vi "MAIN - Create New REx_CMD.vi"() -> ()   [LabVIEW 2012, in "REx_Springboard.lvlib"]
uses:
  _CMD_Springboard/REx_Springboard.lvlib
  _CMD_Springboard/Dependencies.llb/Exit Req Event Registration Ref.ctl
  <vilib>/LabVIEW Icon API/API_Text.ctl
  <vilib>/LabVIEW Icon API/API_User Layer Data.ctl
  <vilib>/Utility/miscctls.llb/LVPoint32TypeDef.ctl
  <vilib>/picture/picture.llb/imagedata.ctl
  <vilib>/LabVIEW Icon API/API_Test Settings.ctl
  <vilib>/LabVIEW Icon API/lv_icon/Controls/Alignment.ctl
  <vilib>/LabVIEW Icon API/API_Text Colors.ctl
  <vilib>/Utility/error.llb/DialogTypeEnum.ctl
  _CMD_Springboard/TypeDef - SHIFTER - GUI Template.ctl
  _CMD_Springboard/Dependencies.llb/TLB_Dependencies.lvlib
  <vilib>/LabVIEW Icon API/LabVIEW Icon API.lvlib
panel:
  out "Icon Preview":picture
  in  "Wait For Response?":bool=TRUE
  in  "Timeout, ms":i32=-1
  in  "Line 2 text":string
  in  "Line 1 text":string
  in  "Add to Project":u16(ring) items=["REx.lvproj", "Untitled Project 1", "< Create In New Project... >"]
  in  "Cancel":bool
  in  "Build":bool
  in  "New Command Name":string
  in  "Destination Folder":path
  out "error out":errorcluster
  # "New REx CMD"
  # "Description"
  # "Configuration"
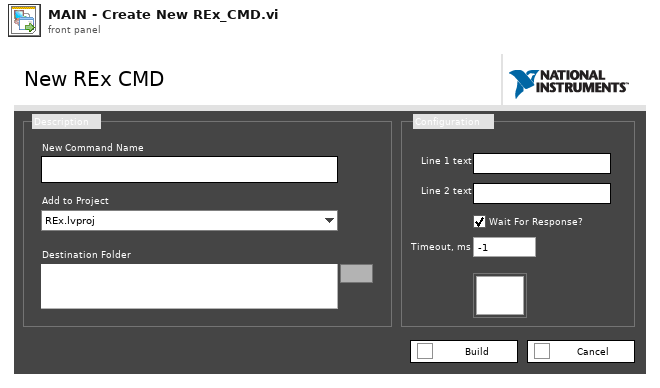
[diagram p1: front panel]
types:
  T1 = enum16{"Clear SR", "Set Display", "Set Shifter", "Initialize Events", "Init Q"}
  T2 = typedef "REx_Springboard.lvlib/TypeDef - SHIFTER - GUI Template.ctl" = cluster{"Exit Event":T3, "Terminate Error":errorcluster, "User Parameter Controls":refnum<vi>[], "User Parameters":cluster{"New REx Name":string, "Destination Folder":path, "Project Selection":u16, "Line 1 text":string, "Line 2 text":string, "Timeout":i32, "Wait For Response?":bool}, "Display Data":cluster{"Copy Successful?":bool}, "Projects In Memory":refnum<vi>[], "New Library Path":path, "Template Library Path":path, "Template Class Reference":refnum<vi>, "Selected Project":refnum<vi>}
  T3 = typedef "REx_Springboard.lvlib/TLB_Dependencies.lvlib/Exit Event Ref.ctl" = refnum<user-event>
  T4 = typedef "REx_Springboard.lvlib/TLB_Dependencies.lvlib/Exit Req Event Registration Ref.ctl" = refnum<event-registration>
  T5 = cluster{"Event Registration Refnum":refnum<event-registration>, "Exit Req Event Registration Ref":T4}
  T6 = typedef "REx_Springboard.lvlib/TLB_Dependencies.lvlib/amc_Message Queue.ctl" = refnum<queue>
  T7 = typedef "LabVIEW Icon API.lvlib/API_User Layer Data.ctl" = cluster{"Layer name":string, "Origin":T8, "Icon image data":T9}
  T8 = typedef "LVPoint32TypeDef.ctl" = cluster{"Horizontal":i32, "Vertical":i32}
  T9 = typedef "imagedata.ctl" = cluster{"image type":i32, "image depth":i32, "image":u8[], "mask":u8[], "colors":u32[], "Rectangle":cluster{"left":i16, "top":i16, "right":i16, "bottom":i16}}
  T10 = typedef "LabVIEW Icon API.lvlib/API_Text.ctl" = cluster{"Line 1 text":string, "Line 2 text":string, "Line 3 text":string, "Line 4 text":string}
  T11 = typedef "DialogTypeEnum.ctl" = enum16{"no dialog", "OK message", "continue or stop message", "auto error handling dialog", "OK message + warnings", "continue/stop + warnings"}
  T12 = typedef "LabVIEW Icon API.lvlib/API_Test Settings.ctl" = cluster{"Font":string, "Alignment":T13, "Size":u8, "Center text":bool, "Capitalize text":bool, "Text color":T14}
  T13 = typedef "Alignment.ctl" = u16
  T14 = typedef "LabVIEW Icon API.lvlib/API_Text Colors.ctl" = cluster{"Line 1 color":u32, "Line 2 color":u32, "Line 3 color":u32, "Line 4 color":u32}
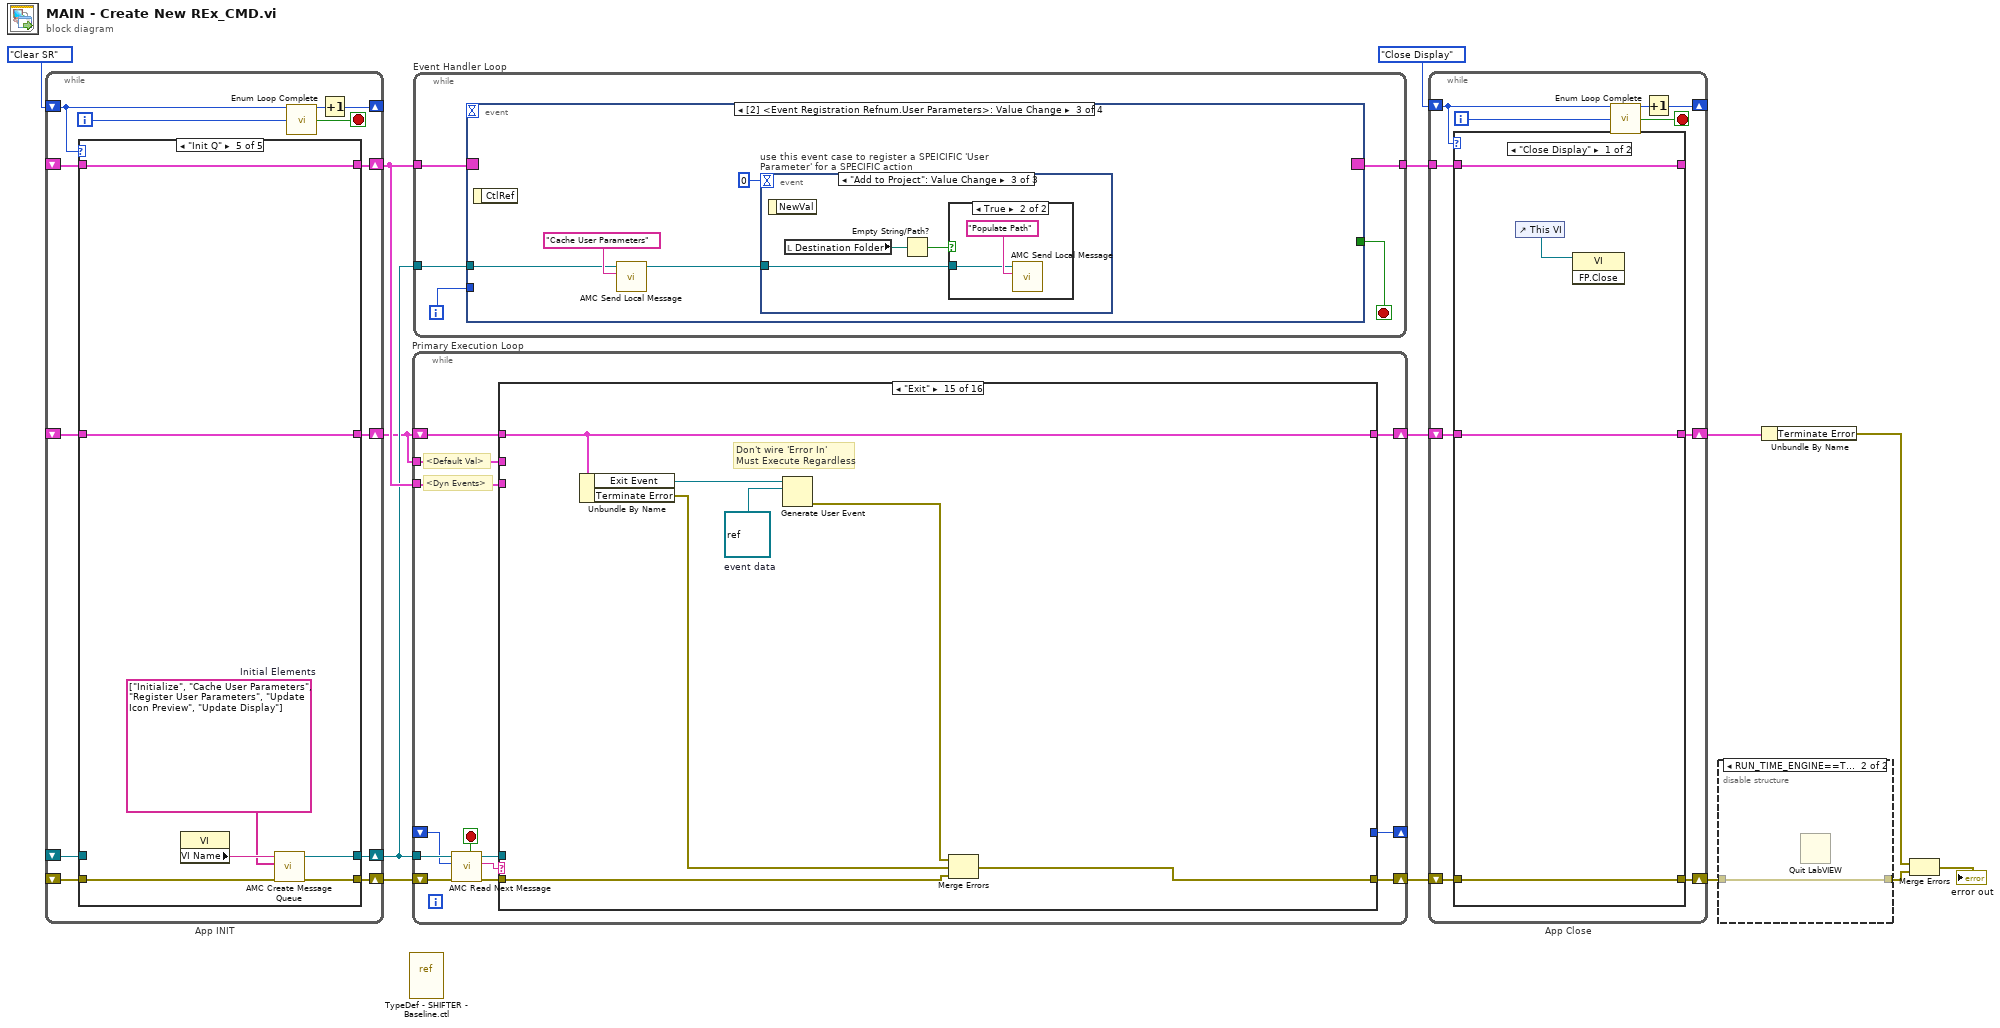
[diagram p0: block diagram]
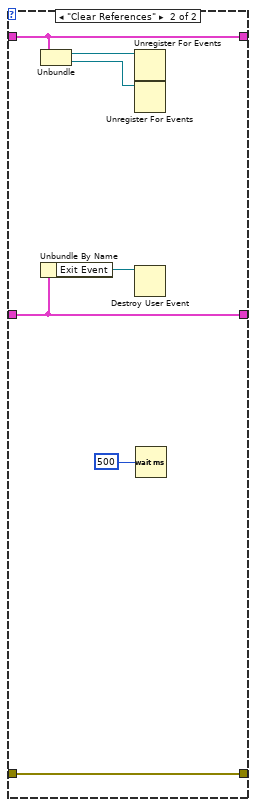
[diagram p3: hidden frame]
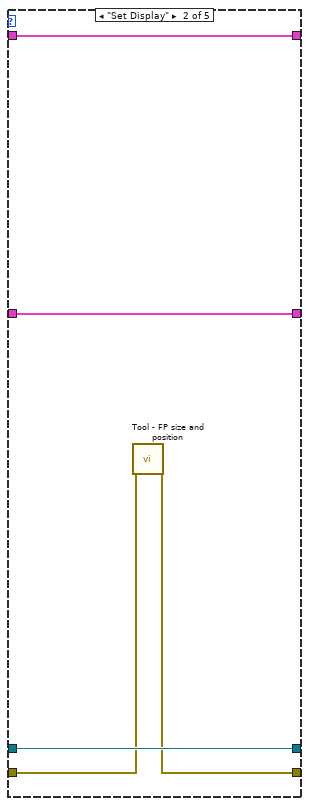
[diagram p5: hidden frame]
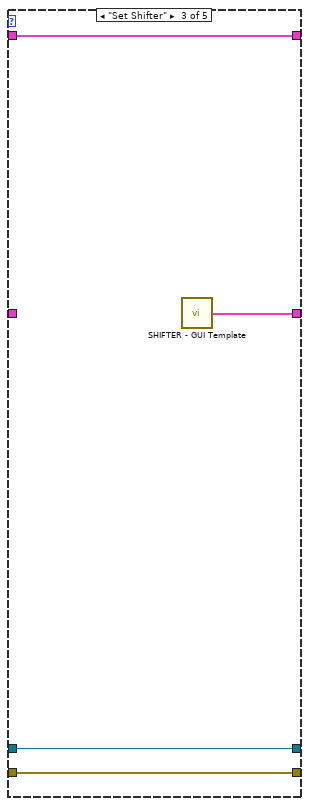
[diagram p6: hidden frame]
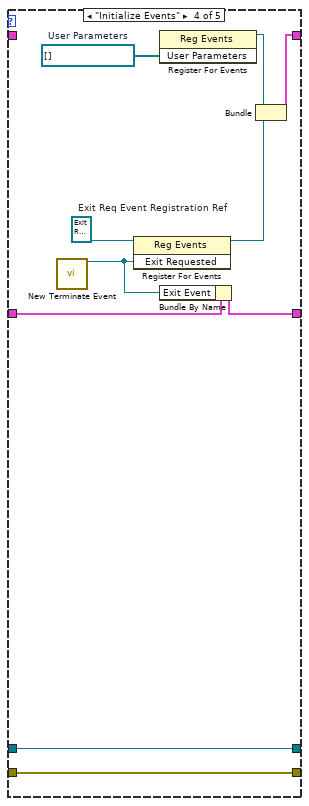
[diagram p7: hidden frame]
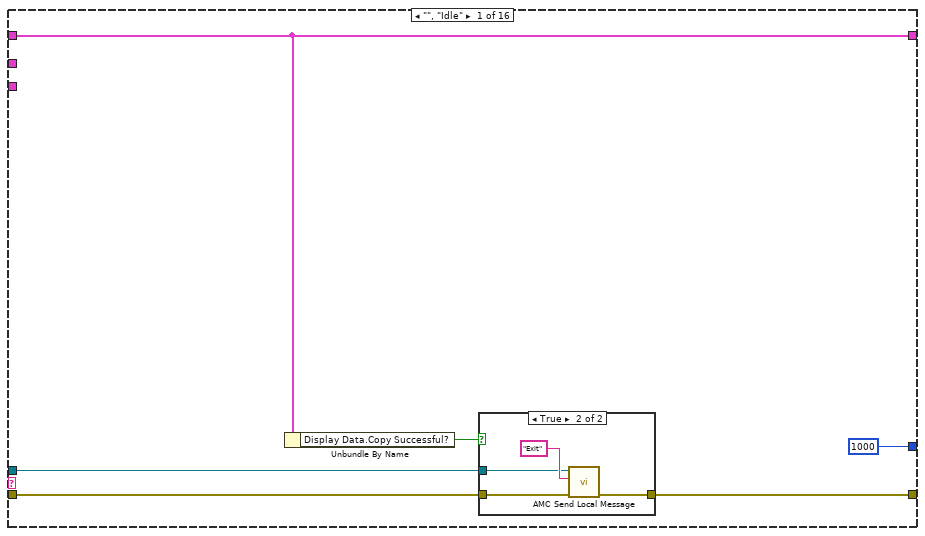
[diagram p8: hidden frame]
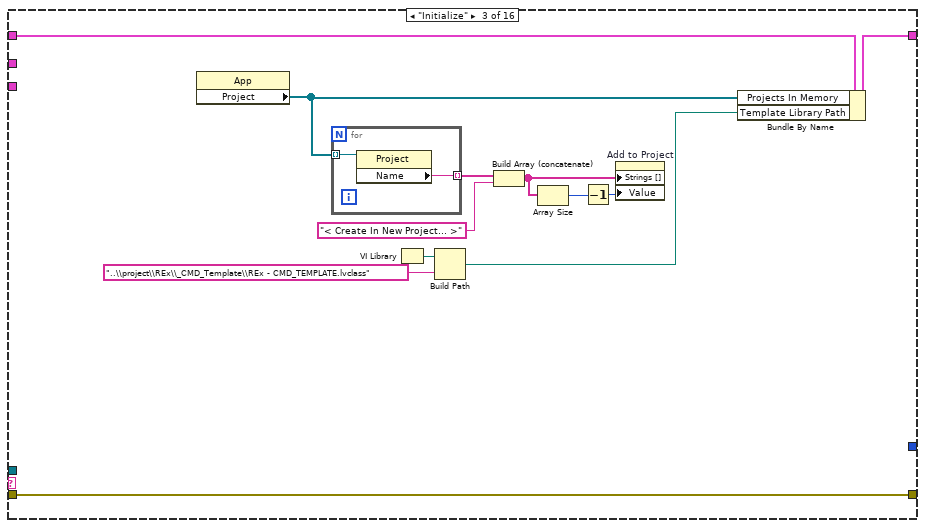
[diagram p11: hidden frame]
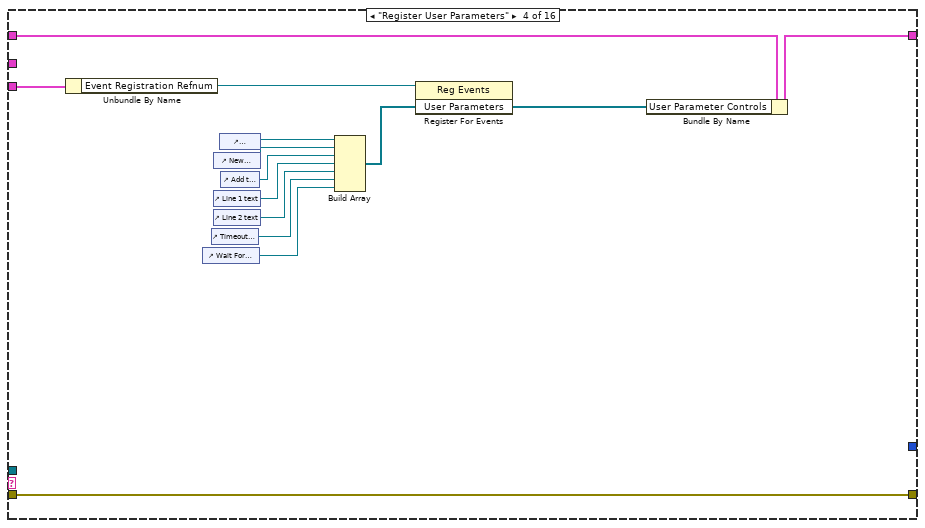
[diagram p12: hidden frame]
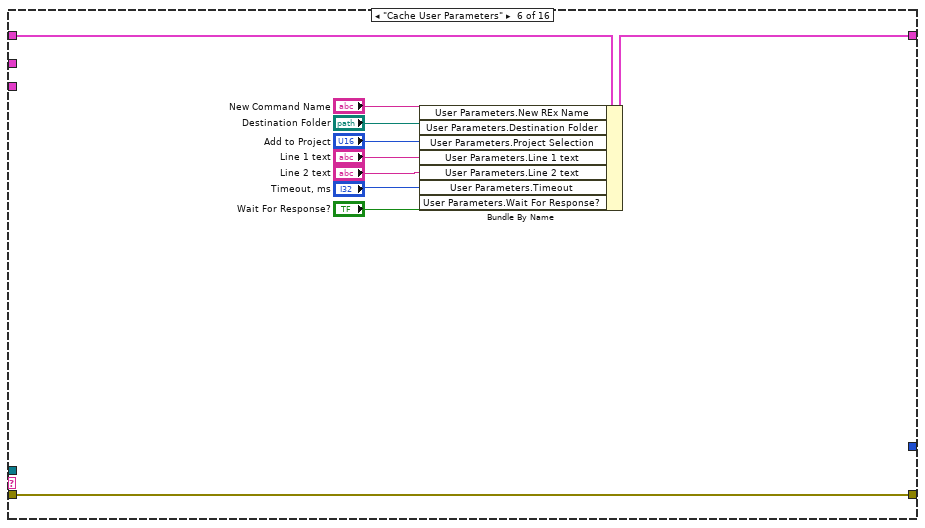
[diagram p14: hidden frame]
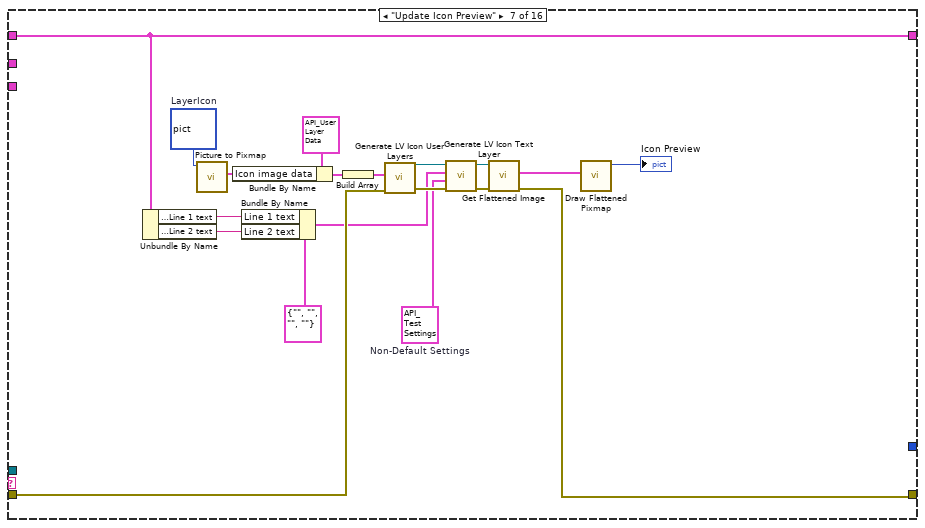
[diagram p15: hidden frame]
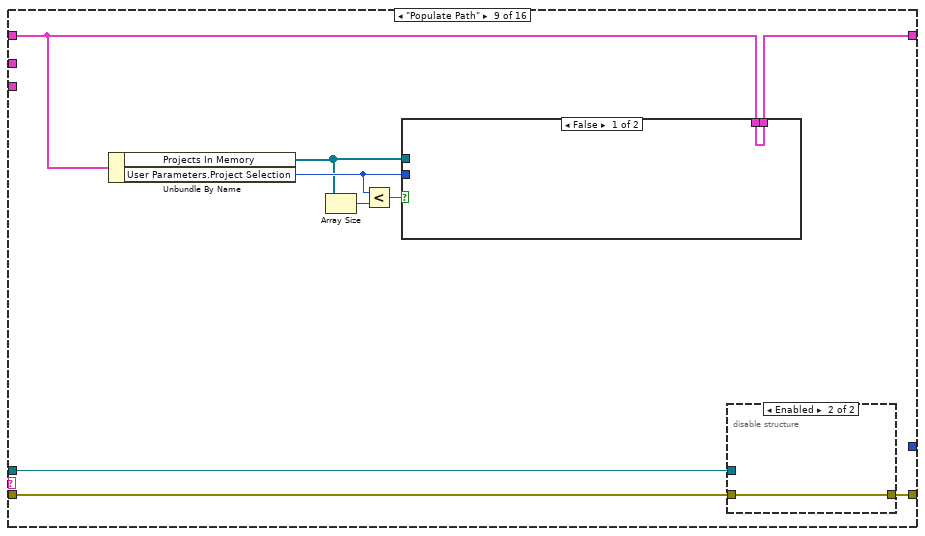
[diagram p17: hidden frame]
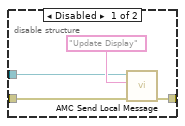
[diagram p18: hidden frame]
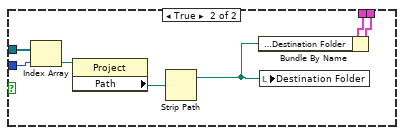
[diagram p19: hidden frame]
diagram:
  n1 = while "App INIT" {
    shift-right: [w20] -> _
    shift-left: T1."Clear SR" -> [w15]
    shift-right: [w26] -> w8
    shift-left: _ -> [w19]
    shift-right: [w23] -> w7
    shift-left: _ -> [w18]
    shift-right: [w25] -> w10
    shift-left: _ -> [w17]
    shift-right: [w24] -> w6
    shift-left: _ -> [w16]
    i -> [w21]
    stop <- w22 stop-if-true
    n2 = case shown="\"Init Q\"" w15 {
      tunnel: [w28 w31 w36 w47 w51] -> w26
      tunnel: [w27 w29 w35 w46 w49] -> w23
      tunnel: [_ w33 w37 w39 w53] -> w24
      tunnel: [_ w32 w34 w44 w54] -> w25
      tunnel: w19 -> [w28 w31 w36 w47 _]
      tunnel: w18 -> [w27 w30 w35 w46 w50]
      tunnel: w17 -> [_ w32 w34 _ w54]
      tunnel: w16 -> [_ w33 _ w40 w53]
      frame "Clear SR" {
      }
      frame "Set Display" {
        n3 = call "Tool - FP size and position.vi"("error in (no error)"=w30) -> ("error out"=w29:errorcluster)  [unwired: 7 in, 11 out]
      }
      frame "Set Shifter" {
        n4 = call "SHIFTER - GUI Template.vi"() -> ("SHIFTER DATA"=w37:T2)  [unwired: 15 out]
      }
      frame "Initialize Events" {
        w41 = T4 refnum  # Exit Req Event Registration Ref
        w45 = refnum<vi>[] []  # User Parameters
        n5 = call "New Terminate Event.vi"() -> ("Exit Event Ref"=w38:T3)  [unwired: 13 in, 2 out]
        n6 = register-events(reference=w41, w38) -> (reference out=w42:T4)  [unwired: 1 in, 1 out]
        n7 = register-events(w45) -> (reference out=w43:refnum<event-registration>)  [unwired: 2 in, 1 out]
        n8 = Bundle By Name(cluster=w40, "Exit Event"=w38) -> (w39:T2)
        n9 = Bundle("Event Registration Refnum"=w43, "Exit Req Event Registration Ref"=w42) -> (w44:T5)  [unwired: 1 in]
      }
      frame "Init Q" {
        w48 = string[] ["Initialize", "Cache User Parameters", "Register User Parameters", "Update Icon Preview", "Update Display"]  # Initial Elements
        n10 = property class="VI"() -> ("VI Name"=w52:string)  [unwired: 2 in, 2 out]
        n11 = call "AMC Create Message Queue.vi"("error in (no error)"=w50, "Initial Message Names"=w48, "Message Queue Name"=w52) -> ("error out"=w49:errorcluster, "Message Queue out"=w51:T6)  [unwired: 7 in]
      }
    }
    n12 = call "Enum Loop Complete.vi"("Current State Enum"=w15, "Itteration"=w21) -> ("Loop Complete?"=w22:bool)  [unwired: 13 out]
    n13 = Increment(x=w15) -> (x+1=w20:T1)
  }
  n14 = vi-ref "TypeDef - SHIFTER - Baseline.ctl"() -> ()  [unwired: 1 out]
  n15 = while "Primary Execution Loop" {
    shift-right: [w67] -> w14
    shift-left: w7 -> [w59]
    shift-right: [w64] -> _
    shift-left: _ -> [w56]
    shift-right: [w63] -> w13
    shift-left: w6 -> [w66]
    tunnel: w6 -> [w65]
    tunnel: w8 -> [w61]
    tunnel: w10 -> [w62]
    stop <- w57 stop-if-true
    # "<Dyn Events>"
    # "<Default Val>"
    n16 = call "AMC Read Next Message.vi"("error in (no error)"=w59, "timeout (1ms)"=w56, "Message Queue in"=w61) -> ("error out"=w58:errorcluster, "Message Name"=w55:string, "Message Queue out"=w60:T6, "Exit Process"=w57:bool)  [unwired: 2 in, 3 out]
    n17 = case shown="\"Exit\"" w55 {
      selector: w55 -> [_ _ _ _ _ _ _ _ _ _ _ _ _ _ _ w237]
      tunnel: [w70 w80 w84 w107 w109 w117 w132 w140 w147 w164 w168 w204 w207 w214 w232 w241] -> w67
      tunnel: w58 -> [w71 w80 w84 w107 w109 w117 w138 w140 w148 w164 w172 w188 w207 w216 w230 w242]
      tunnel: w60 -> [w68 _ _ _ _ _ _ _ w149 _ _ _ _ w212 _ _]
      tunnel: w66 -> [w72 w79 w92 w106 w108 w119 w135 w139 w142 w163 w176 w196 w206 w209 w235 w243]
      tunnel: w65 -> [_ _ _ _ _ _ _ _ _ _ _ _ _ _ _ _]
      tunnel: [w72 w79 w91 w105 w108 w118 w135 w139 w141 w163 w175 w196 w206 w208 w235 w243] -> w63
      tunnel: [1000 _ _ _ _ _ _ _ _ _ _ _ _ _ _ _] -> w64
      tunnel: w62 -> [_ _ _ w104 _ _ _ _ _ _ _ _ _ _ _ _]
      frame "", "Idle" {
        n18 = Unbundle By Name(w72) -> ("Display Data.Copy Successful?"=w69:bool)
        n19 = case shown="True" w69 {
          tunnel: w71 -> [w74 w77]
          tunnel: [w74 w76] -> w70
          tunnel: w68 -> [_ w75]
          frame False {
          }
          frame True {
            n20 = call "AMC Send Local Message.vi"("error in (no error)"=w77, "Message Name"="Exit" ("event"), "Message Queue in"=w75) -> ("error out"=w76:errorcluster)  [unwired: 7 in, 1 out]
          }
        }
      }
      frame "/*********Initialize********/" {
      }
      frame "Initialize" {
        n21 = property class="App"() -> ("Project"=w90:refnum<vi>[])  [unwired: 2 in, 2 out]
        n22 = for {
          tunnel: w90 -> [w94] mode=indexing
          tunnel: [w93] -> w89 mode=indexing
          n23 = property class="Project"(reference=w94) -> ("Name"=w93:string)  [unwired: 1 in, 2 out]
        }
        n24 = VI Library() -> (path=w87:path)
        n25 = Build Path(base path=w87, name or relative path="..\\project\\REx\\_CMD_Template\\REx - CMD_TEMPLATE.lvclass") -> (appended path=w85:path)
        n26 = Build Array (concatenate)(w89, "< Create In New Project... >") -> (w83:string[])
        n27 = Array Size(array=w83) -> (size(s)=w82:i32)
        n28 = Decrement(x=w82) -> (x-1=w81:i32)
        n29 = property on="Add to Project" class="Ring (strict)"("Strings []"=w83, "Value"=w81) -> ()  [unwired: 2 in, 2 out]
        n30 = Bundle By Name(cluster=w92, "Projects In Memory"=w90, "Template Library Path"=w85) -> (w91:T2)
      }
      frame "Register User Parameters" {
        n31 = Unbundle By Name(w104) -> ("Event Registration Refnum"=w103:refnum<event-registration>)
        n32 = control-ref of="Wait For Response?"() -> (w95:refnum<vi>)
        n33 = control-ref of="Timeout, ms"() -> (w96:refnum<vi>)
        n34 = control-ref of="New Command Name"() -> (w99:refnum<vi>)
        n35 = control-ref of="Line 1 text"() -> (w98:refnum<vi>)
        n36 = control-ref of="Line 2 text"() -> (w97:refnum<vi>)
        n37 = control-ref of="Destination Folder"() -> (w102:refnum<vi>)
        n38 = control-ref of="Add to Project"() -> (w100:refnum<vi>)
        n39 = Build Array(w102, w99, w100, w98, w97, w96, w95) -> (w101:refnum<vi>[])
        n40 = register-events(reference=w103, w101) -> ()  [unwired: 1 in, 2 out]
        n41 = Bundle By Name(cluster=w106, "User Parameter Controls"=w101) -> (w105:T2)
      }
      frame "/*********Display Updates********/" {
      }
      frame "Cache User Parameters" {
        n42 = Bundle By Name(cluster=w119, "User Parameters.New REx Name"="New Command Name", "User Parameters.Destination Folder"="Destination Folder", "User Parameters.Project Selection"="Add to Project", "User Parameters.Line 1 text"="Line 1 text", "User Parameters.Line 2 text"="Line 2 text", "User Parameters.Timeout"="Timeout, ms", "User Parameters.Wait For Response?"="Wait For Response?") -> (w118:T2)
      }
      frame "Update Icon Preview" {
        w120 = T12 {"Font"="Small Fonts", "Alignment"=1, "Size"=8, "Center text"=FALSE, "Capitalize text"=TRUE, "Text color"={"Line 1 color"=0, "Line 2 color"=0, "Line 3 color"=0, "Line 4 color"=0}}  # Non-Default Settings
        w127 = picture bytes[3230]  # LayerIcon
        n43 = Unbundle By Name(w135) -> ("User Parameters.Line 1 text"=w137:string, "User Parameters.Line 2 text"=w136:string)
        n44 = call <vilib>:"Picture to Pixmap.vi"("picture"=w127) -> ("image data"=w126:T9)  [unwired: 9 in, 1 out]
        n45 = Bundle By Name(cluster=T7 {"Layer name"="", "Origin"={"Horizontal"=0, "Vertical"=0}, "Icon image data"={"image type"=0, "image depth"=0, "image"=[], "mask"=[], "colors"=[], "Rectangle"={"left"=0, "top"=0, "right"=0, "bottom"=0}}} ("User layer"), "Icon image data"=w126) -> (w125:T7)
        n46 = Bundle By Name(cluster=T10 {"Line 1 text"="", "Line 2 text"="", "Line 3 text"="", "Line 4 text"=""} ("Text"), "Line 1 text"=w137, "Line 2 text"=w136) -> (w121:T10)
        n47 = Build Array(w125) -> (w124:T7[])
        n48 = call <vilib>:"Generate LV Icon User Layers.vi"("error in (no error)"=w138, "User layers"=w124) -> ("error out"=w129:errorcluster, "Icon out"=w123:refnum<class "Icon.lvclass">)  [unwired: 8 in]
        n49 = call <vilib>:"Generate LV Icon Text Layer.vi"("error in (no error)"=w129, "Text settings"=w120, "Text"=w121, "Icon in"=w123) -> ("error out"=w131:errorcluster, "Icon out"=w122:refnum<class "Icon.lvclass">)  [unwired: 6 in]
        n50 = call <vilib>:"Get Flattened Image.vi"("error in (no error)"=w131, "lv_icon.lvlib:Icon.lvclass in"=w122) -> ("error out"=w132:errorcluster, "Color Image"=w134:T9)  [unwired: 6 in, 2 out]
        n51 = call <vilib>:"Draw Flattened Pixmap.vi"("image data"=w134) -> ("new picture"=→"Icon Preview":picture)  [unwired: 8 in]
      }
      frame "Update Display" {
      }
      frame "Populate Path" {
        n52 = Unbundle By Name(w142) -> ("Projects In Memory"=w144:refnum<vi>[], "User Parameters.Project Selection"=w146:u16)
        n53 = Array Size(array=w144) -> (size(s)=w145:i32)
        n54 = Less?(x=w146, y=w145) -> (x < y?=w143:bool)
        n55 = case shown="False" w143 {
          tunnel: w146 -> [_ w162]
          tunnel: w144 -> [_ w161]
          tunnel: w142 -> [w155 w159]
          tunnel: [w155 w158] -> w141
          frame False {
          }
          frame True {
            n56 = Index Array(array=w161, index=w162) -> (element=w160:refnum<vi>)
            n57 = property class="Project"(reference=w160) -> ("Path"=w157:path)  [unwired: 1 in, 2 out]
            n58 = Strip Path(path=w157) -> (stripped path=w156:path)  [unwired: 1 out]
            n59 = Bundle By Name(cluster=w159, "User Parameters.Destination Folder"=w156) -> (w158:T2)
            n60 = local write "Destination Folder"(w156) -> ()
          }
        }
        n61 = disable-structure shown="Enabled" {
          disable-tunnel: w149 -> [w152 _]
          disable-tunnel: w148 -> [w151 w154]
          disable-tunnel: [w150 w154] -> w147
          frame Disabled {
            n62 = call "AMC Send Local Message.vi"("error in (no error)"=w151, "Message Name"="Update Display" ("event"), "Message Queue in"=w152) -> ("error out"=w150:errorcluster)  [unwired: 7 in, 1 out]
          }
          frame Enabled {
          }
        }
      }
      frame "/*********Primary Execution********/" {
      }
      frame "Build New CMD" {
        n63 = Unbundle By Name(w176) -> ("Projects In Memory"=w178:refnum<vi>[], "User Parameters.Project Selection"=w180:u16)
        n64 = Unbundle By Name(w176) -> ("Template Library Path"=w166:path, "User Parameters.Destination Folder"=w171:path, "User Parameters.New REx Name"=w170:string)
        n65 = call <vilib>:"Set Busy.vi"("error in (no error)"=w172) -> ("error out"=w169:errorcluster)  [unwired: 9 in, 1 out]
        n66 = Array Size(array=w178) -> (size(s)=w179:i32)
        n67 = Less?(x=w180, y=w179) -> (x < y?=w177:bool)
        n68 = case shown="True" w177 {
          tunnel: w180 -> [_ w185]
          tunnel: w178 -> [_ w184]
          tunnel: [w181 w183] -> w165
          frame False {
            n69 = invoke class="App" method="Project.New"() -> ("Project:New"=w182:refnum<vi>)  [unwired: 3 in, 2 out]
            n70 = invoke class="Project" method="Open Window"(reference=w182) -> (reference out=w181:refnum<vi>)  [unwired: 2 in, 2 out]
          }
          frame True {
            n71 = Index Array(array=w184, index=w185) -> (element=w183:refnum<vi>)
          }
        }
        n72 = call "Copy Library into Project.vi"("Project"=w165, "Library Path"=w166, "Destination Folder"=w171, "New TLB Name"=w170, "error in"=w169) -> ("New Library Path"=w167:path, "error out"=w168:errorcluster)  [unwired: 9 in]
        n73 = Unbundle By Name(w168) -> ("status"=w174:bool)
        n74 = Not(x=w174) -> (.not. x?=w173:bool)
        n75 = Bundle By Name(cluster=w176, "Display Data.Copy Successful?"=w173, "New Library Path"=w167, "Selected Project"=w165) -> (w175:T2)
      }
      frame "Customize CMD" {
        w201 = refnum<vi> refnum  # LVClassLibrary
        # "*Change Event Terminal Names\n*Change Icon\n*Change Short Name\n*Modify Send Command (Wait / Timeout / Direction of Data"
        n76 = Unbundle By Name(w196) -> ("User Parameters.Line 1 text"=w198:string, "User Parameters.Line 2 text"=w197:string, "User Parameters.New REx Name"=w193:string, "Selected Project"=w186:refnum<vi>)
        n77 = Unbundle By Name(w196) -> ("New Library Path"=w203:path)
        n78 = property class="Project"(reference=w186, error in=w188) -> (error out=w187:errorcluster, "App Ref"=w189:refnum<vi>)  [unwired: 1 out]
        n79 = invoke class="App" method="Library.Open"(reference=w189, error in=w187, "path"=w203) -> (error out=w205:errorcluster, "Open Library"=w202:refnum<vi>)  [unwired: 1 in, 2 out]
        n80 = Unbundle By Name(w196) -> ("User Parameters.Wait For Response?"=w195:bool, "User Parameters.Timeout"=w194:i32)
        n81 = To More Specific Class(target class=w201, reference=w202, error in=w205) -> (specific class reference=w200:refnum<vi>, error out=w199:errorcluster)
        n82 = call "Mutate New CMD.vi"("Class Library in"=w200, "Line 2 text"=w197, "Line 1 text"=w198, "Command name"=w193, "Wait For Response?"=w195, "Timeout"=w194, "error in"=w199) -> ("Class Library out"=w190:refnum<vi>, "error out"=w192:errorcluster)  [unwired: 7 in]
        n83 = Close Reference(reference=w190, error in (no error)=w192) -> (error out=w191:errorcluster)
        n84 = call <vilib>:"Unset Busy.vi"("error in (no error)"=w191) -> ("error out"=w204:errorcluster)  [unwired: 10 in]
      }
      frame "/*********Shutdown********/" {
      }
      frame "Error" {
        n85 = call <vilib>:"General Error Handler CORE.vi"("type of dialog (OK msg:1)"=DialogTypeEnum."auto error handling dialog", "error in (no error)"=w216) -> ("stop event propagated"=w211:bool, "error out"=w215:errorcluster)  [unwired: 12 out]
        n86 = case "User Chose to Stop and Not Continue\nFALSE = Continue: CLEAR ERRORS" shown="False" w211 {
          tunnel: [w227 w228] -> w213
          tunnel: w215 -> [w226 w228]
          frame False {
            n87 = call <vilib>:"Clear Errors.vi"("error in (no error)"=w226) -> ("error out"=w227:errorcluster)  [unwired: 6 out]
          }
          frame True {
          }
        }
        n88 = case "User Chose to Stop and Not Continue" shown="True" w211 {
          tunnel: [w218 w220] -> w214
          tunnel: w213 -> [w218 w222]
          tunnel: w212 -> [_ w219]
          tunnel: w209 -> [w217 w224]
          tunnel: [w217 w223] -> w208
          frame False {
          }
          frame True {
            n89 = call <vilib>:"Clear Errors.vi"("error in (no error)"=w222) -> ("error out"=w221:errorcluster)  [unwired: 6 out]
            n90 = Bundle By Name(cluster=w224, "Terminate Error"=w222) -> (w223:T2)
            n91 = call "AMC Send Local Message.vi"("error in (no error)"=w221, "Message Name"="Exit" ("event"), "Message Queue in"=w219) -> ("error out"=w220:errorcluster)  [unwired: 7 in, 1 out]
          }
        }
      }
      frame "Exit" {
        w229 = refnum<class> refnum  # event data
        # "Don't wire 'Error In'\nMust Execute Regardless"
        n92 = Unbundle By Name(w235) -> ("Exit Event"=w234:T3, "Terminate Error"=w231:errorcluster)
        n93 = Generate User Event(user event=w234, event data cluster=w229) -> (error out=w233:errorcluster)  [unwired: 1 in, 1 out]
        n94 = Merge Errors(w233, w231, w230) -> (w232:errorcluster)
      }
      frame Default {
        w239 = 1 items=["No error", "Argument error", "Memory is full", "Out of zone", "End of file", "File already open", "Generic file I/O error", "File not found", "File permission error", "Disk is full", "Duplicate path", "Too many files open", "System feature not enabled", "Resource file not found", "Cannot add resource", "Resource not found", "Image not found", "Image memory error", "Pen does not exist", "Config type invalid", "Config token not found", "Config parse error", "Config memory error", "Bad external code format", "Bad external code offset", "External code not present", "Null window", "Destroy window error", "Null menu", "Print aborted", "Bad print record", "Print driver error", "Windows error during printing", "Memory error during printing", "Print dialog error", "Generic print error", "Invalid device refnum", "Device not found", "Device parameter error", "Device unit error", "Cannot open device", "Device call aborted", "Generic error", "Cancelled by user", "Object ID too low", "Object ID too high", "Object not in heap", "Unknown heap", "Unknown object (invalid DefProc)", "Unknown object (DefProc not in table)", "Message out of range", "Invalid (null) method", "Unknown message", "Manager call not supported", "Bad address", "Network operation in progress", "Network operation timed out", "Connection is busy", "Network attribute not supported", "Network error", "Address in use", "System out of memory", "Connection aborted", "Connection refused", "Not connected", "Already connected", "Connection closed", "Initialization error (interapplication manager)", "Bad occurrence", "Wait on unbound occurrence handler", "Occurrence queue overflow", "Datalog type conflict", "Unused", "Unrecognized type (interapplication manager)", "Memory corrupt", "Failed to make temporary DLL", "Old CIN version", "Drag socket not found", "Failed to load drop-object", "Failed to register OLE object", "Failed to release OLE object", "Format specifier type mismatch", "Unknown format specifier", "Too few format specifiers", "Too many format specifiers", "Scan failed", "Newer CIN version", "Error converting to variant", "Runtime menu error", "Password tampered", "Variant attribute not found", "Incompatible variant data type", "Event data is not available", "Event Store is not present", "Occurrence is not found", "Event Queue is not created", "Event info is not available", "Refnum passed is NULL", "Error retrieving Class GUID", "Error retrieving CoClass GUID", "Error retrieving TypeLib GUID.", "Bad built application magic bytes.", "Specific driver is different from the specific driver associated with the Logical Name.", "There is no session opened to the class driver.", "Max Error", "MAX - Error with config objects", "MAX - Error loading configuration", "MAX - Group not supported"]
        w240 = TRUE  # status
        n95 = Format Into String(format string="DEVELOPER ERROR:\nImproper State Requested\n================\nState {%s} does not exist within this architecture\n\nCheck for spelling and case errors" ("source"), w237) -> (resulting string=w238:string)  [unwired: 2 in, 1 out]
        n96 = Bundle By Name(cluster=w242, "status"=w240, "code"=w239, "source"=w238) -> (w241:errorcluster)
      }
    }
  }
  n97 = while "Event Handler Loop" {
    tunnel: w10 -> [w247]
    tunnel: w8 -> [w246]
    tunnel: [w245] -> w12
    i -> [w244]
    stop <- w248 stop-if-true
    n98 = event shown="[2] <Event Registration Refnum.User Parameters>: Value Change" {
      selector: w247 -> [_ _ _ _]
      dyn-events: [_ _ _ _] -> w245
      timeout: _ -> [_ _ _ _]
      tunnel: [TRUE ("NewVal") TRUE ("NewVal") _ _] -> w248
      tunnel: w246 -> [w249 w255 w257 w270]
      tunnel: w244 -> [_ _ _ _]
      event Panel Close? {
        w251 = TRUE  # Discard?
        n99 = event-data() -> ()  [unwired: 2 out]
        n100 = call "AMC Send Local Message.vi"("Message Name"="Exit", "Message Queue in"=w249) -> ()  [unwired: 8 in, 2 out]
        n101 = event-data("Discard?"=w251) -> ()  [unwired: 1 in, 1 out]
      }
      event User Event; "Cancel": Value Change {
        n102 = event-data() -> ()  [unwired: 4 out]
        n103 = call "AMC Send Local Message.vi"("Message Name"="Exit", "Message Queue in"=w255) -> ()  [unwired: 8 in, 2 out]
      }
      event Value Change {
        n104 = event-data() -> ()  [unwired: 2 out]
        n105 = call "AMC Send Local Message.vi"("Message Name"="Cache User Parameters" ("event"), "Message Queue in"=w257) -> ("Message Queue out"=w259:T6)  [unwired: 8 in, 1 out]
        n106 = event "use this event case to register a SPEICIFIC 'User Parameter' for a SPECIFIC action" shown="[2] \"Add to Project\": Value Change" {
          selector: _ -> [_ _ _]
          dyn-events: _ -> [_ _ _]
          timeout: 0 -> [_ _ _]
          tunnel: w259 -> [_ w260 w264]
          event Timeout {
            n107 = event-data() -> ()  [unwired: 1 in, 1 out]
          }
          event "Line 1 text", "Line 2 text": Value Change {
            n108 = event-data() -> ()  [unwired: 1 in, 1 out]
            n109 = call "AMC Send Local Message.vi"("Message Name"="Update Icon Preview" ("event"), "Message Queue in"=w260) -> ()  [unwired: 8 in, 2 out]
          }
          event "Add to Project": Value Change {
            n110 = event-data() -> ()  [unwired: 1 in, 1 out]
            n111 = local read "Destination Folder"() -> (w263:path)
            n112 = Empty String/Path?(string/path=w263) -> (empty?=w262:bool)
            n113 = case shown="True" w262 {
              tunnel: w264 -> [_ w265]
              frame False {
              }
              frame True {
                n114 = call "AMC Send Local Message.vi"("Message Name"="Populate Path" ("event"), "Message Queue in"=w265) -> ()  [unwired: 8 in, 2 out]
              }
            }
          }
        }
      }
      event "Build": Value Change {
        n115 = event-data() -> ()  [unwired: 4 out]
        n116 = call "AMC Send Local Message.vi"("Message Name"="Build New CMD" ("event"), "Message Queue in"=w270) -> ("error out"=w267:errorcluster, "Message Queue out"=w268:T6)  [unwired: 8 in]
        n117 = call "AMC Send Local Message.vi"("error in (no error)"=w267, "Message Name"="Customize CMD" ("event"), "Message Queue in"=w268) -> ()  [unwired: 7 in, 2 out]
      }
    }
  }
  n118 = while "App Close" {
    shift-right: [w278] -> _
    shift-left: enum16{"Close Display", "Clear References"}."Close Display" -> [w277]
    tunnel: w12 -> [w275]
    shift-right: [w272] -> w3
    shift-left: w13 -> [w274]
    shift-right: [w273] -> w5
    shift-left: w14 -> [w276]
    i -> [w279]
    stop <- w280 stop-if-true
    n119 = case shown="\"Close Display\"" w277 {
      tunnel: [w282 w291] -> w273
      tunnel: [w284 w287] -> w272
      tunnel: [w283 w290] -> _
      tunnel: w276 -> [w282 w291]
      tunnel: w275 -> [w283 w290]
      tunnel: w274 -> [w284 w287]
      frame "Close Display" {
        n120 = control-ref of="This VI"() -> (w281:refnum<vi>)
        n121 = invoke class="VI" method="FP.Close"(reference=w281) -> ()  [unwired: 2 in, 3 out]
      }
      frame "Clear References" {
        n122 = Unbundle(w290) -> ("Event Registration Refnum"=w289:refnum<event-registration>, "Exit Req Event Registration Ref"=w288:T4)
        n123 = Unbundle By Name(w287) -> ("Exit Event"=w286:T3)
        n124 = Unregister For Events(event registration refnum=w289) -> ()  [unwired: 1 in, 1 out]
        n125 = Unregister For Events(event registration refnum=w288) -> ()  [unwired: 1 in, 1 out]
        n126 = Destroy User Event(user event=w286) -> ()  [unwired: 1 in, 1 out]
        n127 = Wait (ms)(milliseconds to wait=500) -> ()  [unwired: 1 out]
      }
    }
    n128 = call "Enum Loop Complete.vi"("Current State Enum"=w277, "Itteration"=w279) -> ("Loop Complete?"=w280:bool)  [unwired: 13 out]
    n129 = Increment(x=w277) -> (x+1=w278:enum16{"Close Display", "Clear References"})
  }
  n130 = disable-structure shown="RUN_TIME_ENGINE==True" {
    disable-tunnel: [w292 w293] -> w2
    disable-tunnel: w5 -> [w292 w293]
    frame condition #0 (active) {
    }
    frame condition #1 {
      n131 = Quit LabVIEW() -> ()  [unwired: 1 in]
    }
  }
  n132 = Unbundle By Name(w3) -> ("Terminate Error"=w1:errorcluster)
  n133 = Merge Errors(w1, w2) -> (→"error out":errorcluster)
